vi "Set Frequency and Phase.vi"(8 "Error In":errorcluster, 9 "Phase (5 Bit)":u8, 10 "Frequency":u32, 11 "LINX Resource":T1) -> (0 "Error Out":errorcluster, 3 "LINX Resource":T1)   [LabVIEW 2011, in "LVH-LINX.lvlib" / "AD9850.lvlib"]
uses:
  AD9850.lvlib
  Private/Type Defs/LINX Ref.ctl
  Private/Type Defs/Platform.ctl
  Private/Type Defs/Interface.ctl
  Private/Device/Type Defs/LINX Device Config.ctl
  Private/Device/Type Defs/TCP Config.ctl
  Private/Type Defs/Device Family.ctl
  LVH-LINX.lvlib
  Private/Device/Device.lvlib
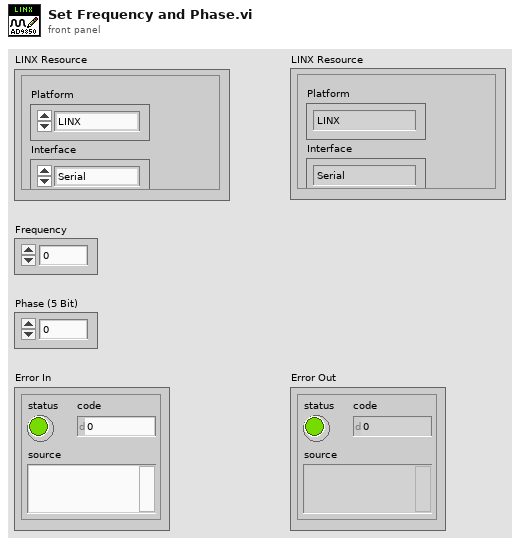
[diagram p1: front panel]
types:
  T1 = typedef "LVH-LINX.lvlib/LINX Ref.ctl" = cluster{"Platform":T2, "Interface":T3, "LINX Device Config":T4}
  T2 = typedef "LVH-LINX.lvlib/Platform.ctl" = enum16{"LINX", "myRIO"}
  T3 = typedef "LVH-LINX.lvlib/Interface.ctl" = enum16{"Serial", "TCP"}
  T4 = typedef "LVH-LINX.lvlib/Device.lvlib/LINX Device Config.ctl" = cluster{"Interface":T3, "COM Port":refnum<visa-resource-name>, "TCP Configuration":T5, "Device Family":T6, "Device ID":u8, "Device Name":string, "TCP Ref":refnum<k5>}
  T5 = typedef "LVH-LINX.lvlib/Device.lvlib/TCP Config.ctl" = cluster{"IP Address":string, "Port":u16}
  T6 = typedef "LVH-LINX.lvlib/Device Family.ctl" = enum8{"National Instruments", "Digilent", "Arduino"}
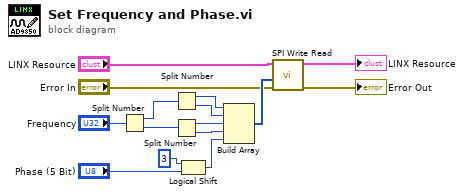
[diagram p0: block diagram]
diagram:
  n1 = Split Number(x="Frequency") -> (hi(x)=w12:u16, lo(x)=w11:u16)
  n2 = Split Number(x=w12) -> (hi(x)=w14:u8, lo(x)=w13:u8)
  n3 = Split Number(x=w11) -> (hi(x)=w10:u8, lo(x)=w9:u8)
  n4 = Logical Shift(y=i8 3, x="Phase (5 Bit)") -> (x << y=w6:u8)
  n5 = Build Array(w14, w13, w10, w9, w6) -> (w5:u8[])
  n6 = call "SPI Write Read.vi"("Error In"="Error In", "Data"=w5, "LINX Resource"="LINX Resource") -> ("Error Out"=→"Error Out":errorcluster, "LINX Resource"=→"LINX Resource":T1)  [unwired: 6 in, 1 out]
